vi "calculateTriggerTimes.vi"(9 "Current time":timestamp, 10 "Record length* (s)":dbl, 11 "Pre-trigger time* (s)":dbl) -> (3 "Trigger timestamps":T1)   [LabVIEW 2017]
doc: "Take in the current time, the amount of pre-trigger time, and the recording length, and generate a trigger timestamp cluster."
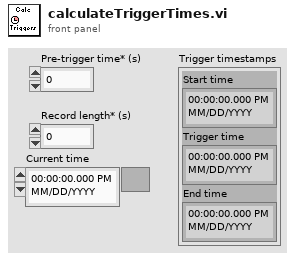
[diagram p1: front panel]
types:
  T1 = cluster{"Start time":timestamp, "Trigger time":timestamp, "End time":timestamp}
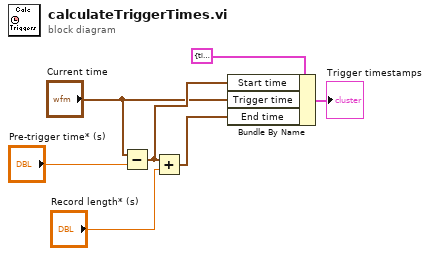
[diagram p0: block diagram]
diagram:
  n1 = Subtract(x="Current time", y="Pre-trigger time* (s)") -> (x-y=w5:timestamp)
  n2 = Add(x=w5, y="Record length* (s)") -> (x+y=w7:timestamp)
  n3 = Bundle By Name(cluster=T1 {"Start time"=timestamp(0 s since 1904-01-01), "Trigger time"=timestamp(0 s since 1904-01-01), "End time"=timestamp(0 s since 1904-01-01)} ("element"), "Start time"=w5, "Trigger time"="Current time", "End time"=w7) -> (→"Trigger timestamps":T1)
